vi "whisker_ccd.vi"() -> ()   [LabVIEW 2019]
panel:
  out "Numeric":i32
  in  "Trigger":bool=TRUE
  in  "Color vs Monochrome":string="Y800 (720x540)"
  in  "ICImagingControl":refnum<k7>(container)
  out "Image":T1(plugin-control)
  in  "AVI Path":path=path "D:/Haad/v1.avi"
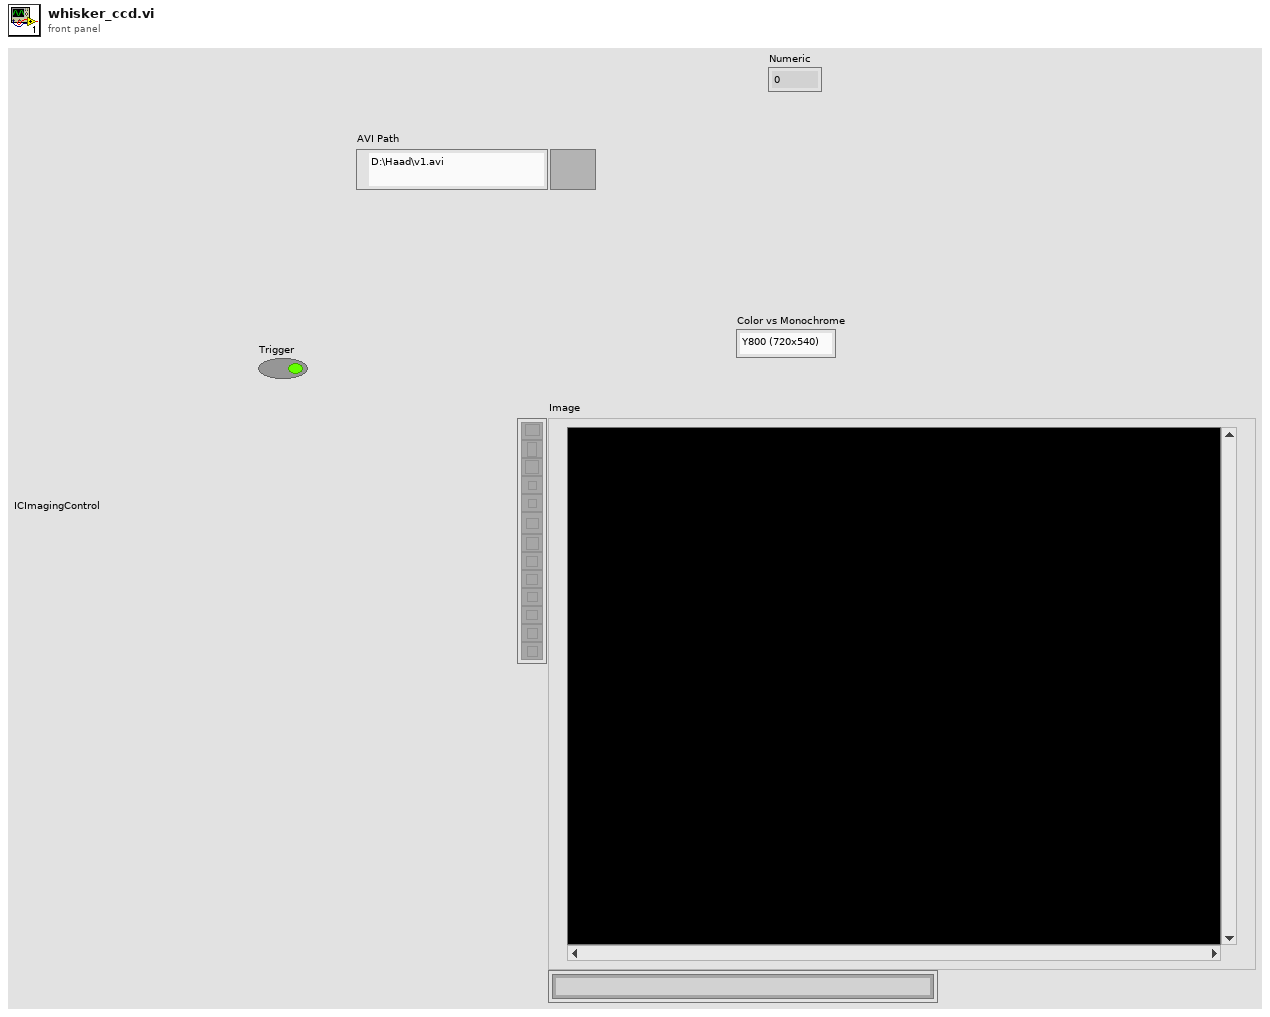
[diagram p1: front panel]
types:
  T1 = typedef "IMAQ Image.ctl" = refnum<image>
  T2 = typedef "IMAQ AVI2 Refnum.ctl" = refnum<k20>
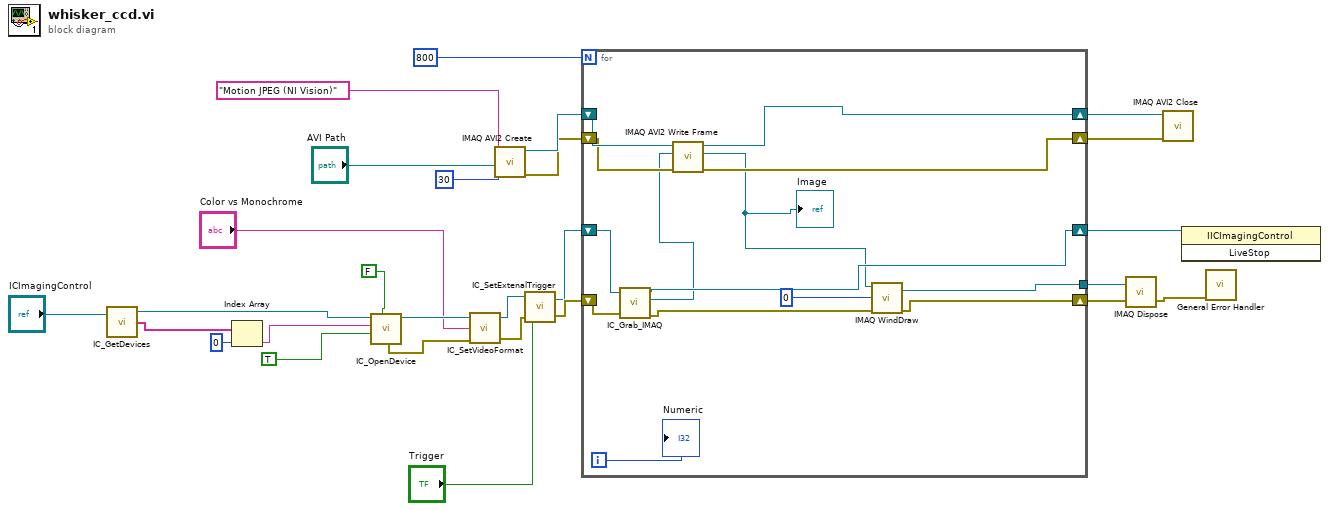
[diagram p0: block diagram]
diagram:
  n1 = call <userlib>:"IC_GetDevices.vi"("ICImagingControl In"="ICImagingControl") -> ("ICImagingControl Out"=w17:refnum<k7>, "Devices"=w16:string[])  [unwired: 1 in, 1 out]
  n2 = Index Array(array=w16, index=0) -> (element=w14:string)
  n3 = call <userlib>:"IC_OpenDevice.vi"("Color"=FALSE, "Live"=TRUE, "Device"=w14, "ICImagingControl In"=w17) -> ("ICImagingControl Out"=w9:refnum<k7>, "Error Out"=w7:errorcluster)  [unwired: 2 in, 4 out]
  n4 = call <userlib>:"IC_SetVideoFormat.vi"("Error In (no error)"=w7, "VideoFormat"="Color vs Monochrome", "ICImagingControl In"=w9) -> ("Error Out"=w4:errorcluster, "ICImagingControl Out"=w6:refnum<k7>)  [unwired: 1 out]
  n5 = call "IMAQ AVI2 Create"("Codec"="Motion JPEG (NI Vision)", "Frames Per Second"=u32 30, "AVI Path"="AVI Path") -> ("error out"=w22:errorcluster, "AVI Refnum"=w25:T2)  [unwired: 7 in]
  n6 = call <userlib>:"IC_SetExtenalTrigger.vi"("Error In (no error)"=w4, "Trigger"="Trigger", "ICImagingControl In"=w6) -> ("Error Out"=w3:errorcluster, "ICImagingControl Out"=w2:refnum<k7>)
  n7 = for {
    N: 800 -> [_]
    tunnel: [w37] -> w13
    shift-right: [w40] -> w24
    shift-left: w25 -> [w41]
    shift-right: [w39] -> w23
    shift-left: w22 -> [w38]
    shift-right: [w36] -> w12
    shift-left: w3 -> [w34]
    shift-right: [w35] -> w10
    shift-left: w2 -> [w33]
    i -> [w28]
    n8 = call <userlib>:"IC_Grab_IMAQ.vi"("ICImagingControl In"=w33, "Error In (no error)"=w34) -> ("ICImagingControl Out"=w35:refnum<k7>, "Image Out"=w30:T1, "Error Out"=w31:errorcluster)  [unwired: 1 in, 1 out]
    n9 = call "IMAQ AVI2 Write Frame"("error in (no error)"=w38, "Image"=w30, "AVI Refnum"=w41) -> ("error out"=w39:errorcluster, "Image Out (duplicate)"=w29:T1, "AVI Refnum (duplicate)"=w40:T2)  [unwired: 6 in]
    "Image" <- w29
    n10 = call "IMAQ WindDraw"("Window Number (0...15)"=0, "error in (no error)"=w31, "Image"=w29) -> ("error out"=w36:errorcluster, "Image Out (duplicate)"=w37:T1)  [unwired: 7 in]
    "Numeric" <- w28
  }
  n11 = call "IMAQ Dispose"("Image"=w13, "error in (no error)"=w12) -> ("error out"=w11:errorcluster)  [unwired: 4 in]
  n12 = call "IMAQ AVI2 Close"("error in (no error)"=w23, "AVI Refnum"=w24) -> ()  [unwired: 9 in, 1 out]
  n13 = invoke class="IICImagingControl" method="LiveStop"(reference=w10) -> ()  [unwired: 2 in, 3 out]
  n14 = call <vilib>:"General Error Handler.vi"("error in (no error)"=w11) -> ()  [unwired: 10 in, 5 out]
